vi "BuildPacket.vi"(1 "Phase Mode":i16, 2 "Tank 2":u16, 3 "Tank 1":u16) -> (0 "PacketArray":i32[](array[numeric]))   [LabVIEW 2011]
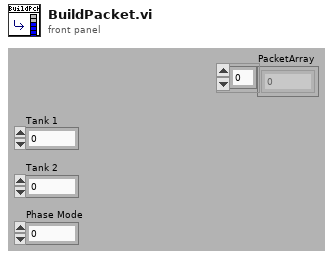
[diagram p1: front panel]
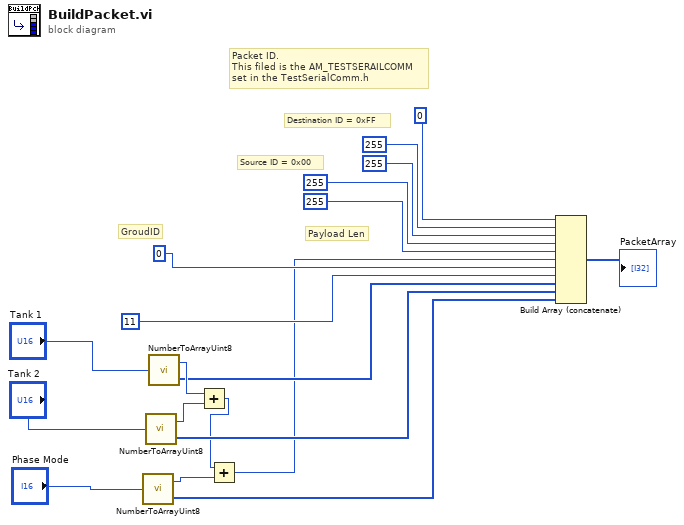
[diagram p0: block diagram]
diagram:
  # "Packet ID.\nThis filed is the AM_TESTSERAILCOMM \nset in the TestSerialComm.h"
  # "GroudID"
  # "Payload Len"
  # "Source ID = 0x00"
  # "Destination ID = 0xFF"
  n1 = call "NumberToArrayUint8.vi"("Numeric 2"="Phase Mode") -> ("Array"=w5:i8[], "Numeric"=w4:i32)
  n2 = call "NumberToArrayUint8.vi"("Numeric 2"="Tank 2") -> ("Array"=w15:i8[], "Numeric"=w17:i32)
  n3 = call "NumberToArrayUint8.vi"("Numeric 2"="Tank 1") -> ("Array"=w14:i8[], "Numeric"=w16:i32)
  n4 = Add(x=w16, y=w17) -> (x+y=w3:i32)
  n5 = Add(x=w3, y=w4) -> (x+y=w2:i32)
  n6 = Build Array (concatenate)(0, 255, 255, 255, 255, w2, 0, i8 11, w14, w15, w5) -> (→"PacketArray":i32[])
